vi "Config - TransferMaster2Slave.vi"(8 "Fehler (Eingang, kein Fehler)":errorcluster, 11 "Devices":cluster{"UartIndex":i32, "Address":i32}[](array[cluster])) -> (0 "Fehler (Ausgang)":errorcluster)   [LabVIEW 2016]
uses:
  GantnerDLL/eGateUtility.dll
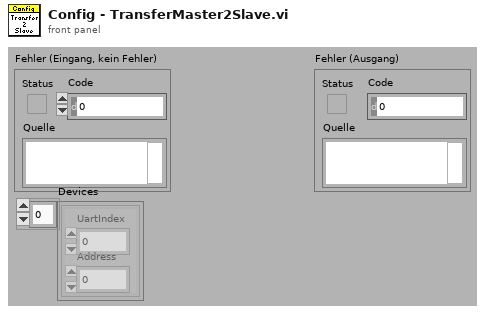
[diagram p1: front panel]
types:
  T1 = enum16{"open", "replace", "create", "open or create", "replace or create", "replace or create with confirmation"}
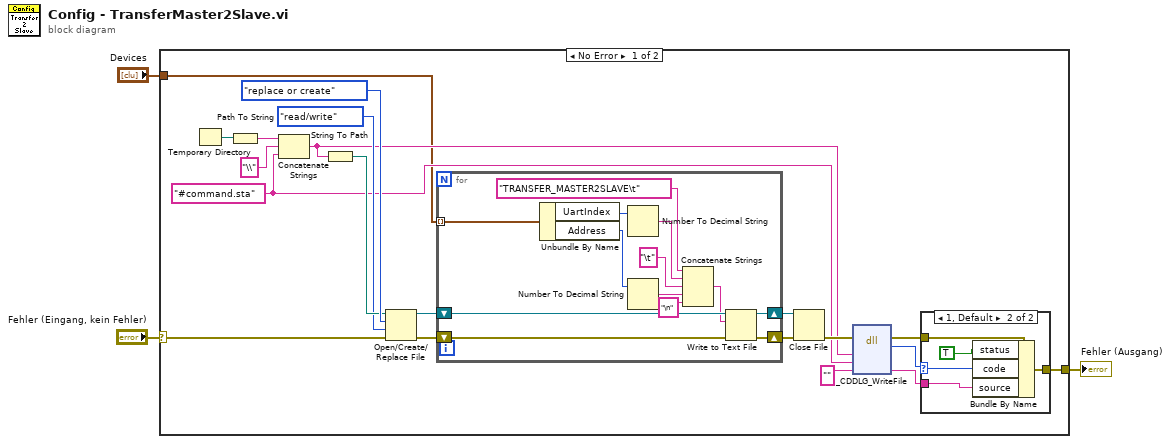
[diagram p0: block diagram]
diagram:
  n1 = case shown="No Error" "Fehler (Eingang, kein Fehler)" {
    selector: "Fehler (Eingang, kein Fehler)" -> [w13 w43]
    tunnel: [w11 w43] -> w2
    tunnel: "Devices" -> [w4 _]
    frame No Error {
      w17 = "#command.sta" ("String")
      n2 = Temporary Directory() -> (w15:path)
      n3 = Path To String(path=w15) -> (string=w14:string)
      n4 = Concatenate Strings(w14, "\\" ("String"), w17) -> (w18:string)
      n5 = String To Path(string=w18) -> (path=w21:path)
      n6 = Open/Create/Replace File(file path (use dialog)=w21, error in=w13, operation (0:open)=T1."replace or create" ("Operation (0:Öffnen)"), access (0:read/write)=enum16{"read/write", "read-only", "write-only"}."read/write" ("Zugriff (0:Lesen/Schreiben)")) -> (refnum out=w8:refnum<file>, error out=w6:errorcluster)  [unwired: 3 out]
      n7 = for {
        shift-right: [w35] -> w7
        shift-left: w8 -> [w36]
        shift-right: [w33] -> w5
        shift-left: w6 -> [w34]
        tunnel: w4 -> [w32] mode=indexing
        n8 = Unbundle By Name(w32) -> ("UartIndex"=w30:i32, "Address"=w27:i32)
        n9 = Number To Decimal String(number=w30) -> (decimal integer string=w29:string)  [unwired: 1 out]
        n10 = Number To Decimal String(number=w27) -> (decimal integer string=w26:string)  [unwired: 1 out]
        n11 = Concatenate Strings("TRANSFER_MASTER2SLAVE\t" ("String"), w29, "\t" ("String"), w26, "\n" ("String")) -> (w25:string)
        n12 = Write to Text File(file (use dialog)=w36, text=w25, error in=w34) -> (refnum out=w35:refnum<file>, error out=w33:errorcluster)  [unwired: 2 out]
      }
      n13 = Close File(refnum=w7, error in=w5) -> (error out=w19:errorcluster)  [unwired: 1 out]
      n14 = dll-call lib="PTH2abs E00. ç³»ç»éæ$17S007 11æ-Gantnerééå°-ç§¦é·SourceCodesHardWareGantner\nGantnerDriver\nGantnerDLLeGateUtility.dll" fn="_CDDLG_WriteFile"(error in=w19, "SourceFullFileName"=w18, "DestinationFileName"=w17, "ErrorString"="") -> (error out=w12:errorcluster, "Rückgabetyp"=w9:i32, "ErrorString"=w10:string)  [unwired: 3 in, 2 out]
      n15 = case shown="1, Default" w9 {
        selector: w9 -> [_ w40]
        tunnel: w12 -> [w37 w42]
        tunnel: [w37 w41] -> w11
        tunnel: w10 -> [_ w38]
        frame 0 {
        }
        frame 1, Default {
          n16 = Bundle By Name(cluster=w42, "status"=TRUE, "code"=w40, "source"=w38) -> (w41:errorcluster)
        }
      }
    }
    frame Error {
    }
  }
  "Fehler (Ausgang)" <- w2
